vi "p2.vi"() -> ()   [LabVIEW 2025, in "d10.lvlib"]
uses:
  d10.lvlib
  lv2025-aoc/AOC/AOC.lvlib
  <vilib>/gmath/NI_Gmath.lvlib
panel:
  out "Answer":i64
  in  "Example":string="[.##.] (3) (1,3) (2) (2,3) (0,2) (0,1) {3,5,4,7}\n[...#.] (0,2,3,4) (2,3) (0,4) (0,1,2) (1,2,3,4) {7,5,12,7,2}\n[.###.#] (0,1,2,3,4) (0,3,4) (0,1,2,4,5) (1,2) {10,11,11,5,10,5}"
  in  "Example 2":bool=TRUE
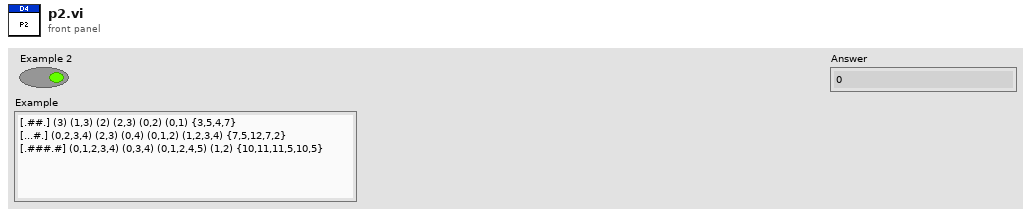
[diagram p1: front panel]
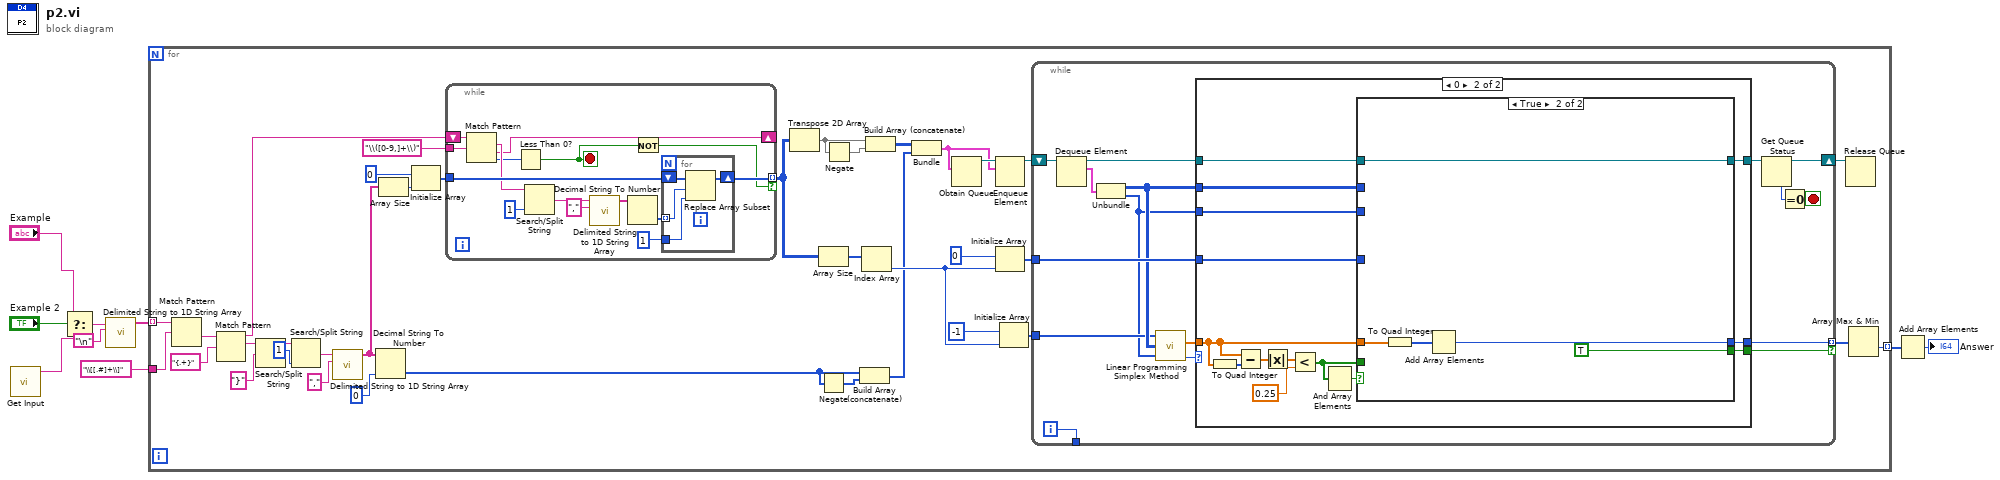
[diagram p0: block diagram]
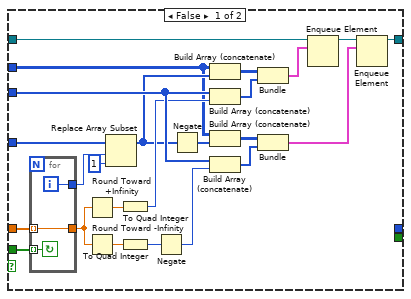
[diagram p3: hidden frame]
diagram:
  n1 = call "Get Input.vi"() -> ("Input"=w9:string)  [unwired: 11 in]
  n2 = Select(t="Example", s="Example 2", f=w9) -> (s? t:f=w3:string)
  n3 = call <vilib>:"Delimited String to 1D String Array.vi"("delimiter"="\n", "delimited string"=w3) -> ("string array"=w5:string[])  [unwired: 9 in]
  n4 = for {
    tunnel: w5 -> [w45] mode=indexing
    tunnel: [w12] -> w2 mode=indexing
    tunnel: "\\[[.#]+\\]" ("regular expression") -> [w10]
    n5 = Match Pattern(string=w45, regular expression=w10) -> (after substring=w44:string)  [unwired: 1 in, 3 out]
    n6 = Match Pattern(string=w44, regular expression="{.+}") -> (before substring=w42:string, match substring=w37:string)  [unwired: 1 in, 2 out]
    n7 = Search/Split String(string=w37, search string/char (-)="}") -> (substring before match=w41:string)  [unwired: 1 in, 2 out]
    n8 = Search/Split String(string=w41, offset (0)=1) -> (match + rest of string=w34:string)  [unwired: 1 in, 2 out]
    n9 = call <vilib>:"Delimited String to 1D String Array.vi"("delimiter"=",", "delimited string"=w34) -> ("string array"=w35:string[])  [unwired: 9 in]
    n10 = Decimal String To Number(string=w35, default (0L)=i64 0 ("default (0 I32)")) -> (number=w15:i64[])  [unwired: 1 in, 1 out]
    n11 = Array Size(array=w35) -> (size(s)=w32:i32)
    n12 = Initialize Array(i64 0 ("default (0 I32)"), w32) -> (w30:i64[])
    n13 = while {
      shift-right: [w113] -> _
      shift-left: w42 -> [w116]
      tunnel: w30 -> [w122]
      tunnel: [w117] -> w29 mode=indexing if=w109
      tunnel: "\\([0-9,]+\\)" ("regular expression") -> [w115]
      stop <- w110 stop-if-true
      n14 = Match Pattern(string=w116, regular expression=w115) -> (match substring=w114:string, after substring=w113:string, offset past match=w111:i32)  [unwired: 1 in, 1 out]
      n15 = Less Than 0?(x=w111) -> (x < 0?=w110:bool)
      n16 = Search/Split String(string=w114, offset (0)=1) -> (match + rest of string=w118:string)  [unwired: 1 in, 2 out]
      n17 = call <vilib>:"Delimited String to 1D String Array.vi"("delimiter"=",", "delimited string"=w118) -> ("string array"=w121:string[])  [unwired: 9 in]
      n18 = Decimal String To Number(string=w121) -> (number=w120:i32[])  [unwired: 2 in, 1 out]
      n19 = Not(x=w110) -> (.not. x?=w109:bool)
      n20 = for {
        shift-right: [w125] -> w117
        shift-left: w122 -> [w127]
        tunnel: w120 -> [w126] mode=indexing
        tunnel: u64 1 ("offset (0)") -> [w124]
        n21 = Replace Array Subset(array=w127, new element=w124, index=w126) -> (w125:i64[])
      }
    }
    n22 = Transpose 2D Array(2D array=w29) -> (transposed array=w19:i64[][])
    n23 = Array Size(array=w29) -> (size(s)=w31:i32[])
    n24 = Negate(x=w15) -> (-x=w16:i64[])
    n25 = Negate(x=w19) -> (-x=w17:i64[][])
    n26 = Build Array (concatenate)(w15, w16) -> (w14:i64[])
    n27 = Index Array(array=w31) -> (element=w21:i32)  [unwired: 1 in]
    n28 = Build Array (concatenate)(w19, w17) -> (w18:i64[][])
    n29 = Bundle(w18, w14) -> (w26:cluster{i64[][], i64[]})  [unwired: 1 in]
    n30 = Obtain Queue(element data type=w26) -> (queue out=w28:refnum<queue>)  [unwired: 4 in, 2 out]
    n31 = Enqueue Element(queue=w28, element=w26) -> (queue out=w27:refnum<queue>)  [unwired: 2 in, 2 out]
    n32 = Initialize Array(i64 0 ("element"), w21) -> (w20:i64[])
    n33 = Initialize Array(i64 -1 ("offset (0)"), w21) -> (w23:i64[])
    n34 = while {
      tunnel: w20 -> [w60]
      shift-right: [w53] -> w24
      shift-left: w27 -> [w59]
      tunnel: [w54] -> w13 mode=indexing if=w47
      tunnel: [w50] -> _
      tunnel: w23 -> [w49]
      i -> [w50]
      stop <- w46 stop-if-true
      n35 = Dequeue Element(queue=w59) -> (queue out=w57:refnum<queue>, element=w58:cluster{i64[][], i64[]})  [unwired: 2 in, 2 out]
      n36 = Unbundle(w58) -> (w55:i64[][], w48:i64[])
      n37 = call <vilib>:"Linear Programming Simplex Method.vi"("C"=w49, "M"=w55, "B"=w48) -> ("X"=w61:dbl[], "error"=w51:i32)  [unwired: 2 out]
      n38 = case shown="0" w51 {
        tunnel: w61 -> [_ w67]
        tunnel: w60 -> [_ w75]
        tunnel: w48 -> [_ w74]
        tunnel: w57 -> [w62 w73]
        tunnel: [w62 w72] -> w56
        tunnel: [_ w71] -> w54
        tunnel: w55 -> [_ w66]
        tunnel: [_ w64] -> w47
        frame Default {
        }
        frame 0 {
          n39 = To Quad Integer(1:w67) -> (0:w70:i64[])
          n40 = Subtract(x=w67, y=w70) -> (x-y=w69:dbl[])
          n41 = Absolute Value(x=w69) -> (abs(x)=w68:dbl[])
          n42 = Less?(x=w68, y=0.25) -> (x < y?=w63:bool[])
          n43 = And Array Elements(Boolean array=w63) -> (logical AND=w65:bool)
          n44 = case shown="True" w65 {
            tunnel: w63 -> [w100 _]
            tunnel: w67 -> [w99 w106]
            tunnel: w75 -> [w98 _]
            tunnel: w74 -> [w91 _]
            tunnel: w73 -> [w87 w108]
            tunnel: [w84 w108] -> w72
            tunnel: [_ w107] -> w71
            tunnel: w66 -> [w79 _]
            tunnel: [_ TRUE] -> w64
            frame False {
              n45 = for {
                tunnel: w100 -> [w103] mode=indexing
                tunnel: w99 -> [w102] mode=indexing
                tunnel: [w102] -> w96
                tunnel: [w101] -> w94
                i -> [w101]
                stop <- w103 continue-if-true
              }
              n46 = Round Toward +Infinity(x=w96) -> (ceil(x): smallest int >= x=w95:dbl)
              n47 = Round Toward -Infinity(1:w96) -> (0:w93:dbl)
              n48 = Replace Array Subset(array=w98, new element=i64 1 ("new element/subarray"), index=w94) -> (w81:i64[])
              n49 = To Quad Integer(1:w95) -> (0:w82:i64)
              n50 = To Quad Integer(1:w93) -> (0:w92:i64)
              n51 = Negate(x=w92) -> (-x=w80:i64)
              n52 = Negate(x=w81) -> (-x=w77:i64[])
              n53 = Build Array (concatenate)(w79, w81) -> (w78:i64[][])
              n54 = Build Array (concatenate)(w91, w82) -> (w90:i64[])
              n55 = Build Array (concatenate)(w79, w77) -> (w88:i64[][])
              n56 = Build Array (concatenate)(w91, w80) -> (w89:i64[])
              n57 = Bundle(w78, w90) -> (w86:cluster{i64[][], i64[]})  [unwired: 1 in]
              n58 = Bundle(w88, w89) -> (w83:cluster{i64[][], i64[]})  [unwired: 1 in]
              n59 = Enqueue Element(queue=w87, element=w86) -> (queue out=w85:refnum<queue>)  [unwired: 2 in, 2 out]
              n60 = Enqueue Element(queue=w85, element=w83) -> (queue out=w84:refnum<queue>)  [unwired: 2 in, 2 out]
            }
            frame True {
              n61 = To Quad Integer(1:w106) -> (0:w105:i64[])
              n62 = Add Array Elements(numeric array=w105) -> (sum=w107:i64)
            }
          }
        }
      }
      n63 = Get Queue Status(queue=w56) -> (queue out=w53:refnum<queue>, # elements in queue=w52:i32)  [unwired: 2 in, 6 out]
      n64 = Equal To 0?(x=w52) -> (x = 0?=w46:bool)
    }
    n65 = Release Queue(queue=w24) -> ()  [unwired: 2 in, 3 out]
    n66 = Array Max & Min(array=w13) -> (min value=w12:i64)  [unwired: 3 out]
  }
  n67 = Add Array Elements(numeric array=w2) -> (sum=→"Answer":i64)
